vi "Measurement UI.vi"() -> ()   [LabVIEW 2021, in "Load Transient_Channel Ganging_UI.lvlib"]
uses:
  Load Transient_Channel Ganging_UI.lvlib
panel:
  in  "MeasGraphs":T1(tab)
  out "OutputCurrentV/STimeGraph":waveform(dbl)(graph) caption="Load Transient"
  in  "Load Current v/s Time":string="LOAD CURRENT vs TIME"
  in  "Output Voltage v/s Time":string="LOAD VOLTAGE vs TIME"
  out "OutputVoltageV/STimeGraph":waveform(dbl)(graph) caption="Load Transient"
  out "dt":dbl
  in  "Load current pole-zero ratio":dbl=0.3
  in  "Load current compensation frequency":dbl=180000.0
  in  "Load current gain bandwidth":dbl=14000.0
  in  "Source voltage pole-zero ratio":dbl=2.0
  in  "Source voltage compensation frequency":dbl=3530.0
  in  "Source voltage gain bandwidth":dbl=2000.0
  out "Ganged load voltages":dbl[](array[numeric])
  out "Ganged load current":dbl[](array[numeric])
  in  "Load slave resource names":string[](array[string])
  in  "Load master resource name":string
  in  "Source slave resource names":string[](array[string])
  in  "Source master resource name":string
  in  "MeasConfigurations":T2(tab)=enum."Source Config"
  in  "Nominal output voltage":dbl=1.0 caption="NOMINAL OUTPUT VOLTAGE" format="%.3pV"
  in  "DUT setup time":dbl=1.0 caption="DUT SETUP TIME" format="%.3ps"
  in  "Level dwell time":dbl=0.001 caption="DWELL TIME" format="%.3ps"
  in  "PPSSlaveResourceNames":refnum<k15>[](array[refnum]) caption="SLAVE RESOURCE NAMES"
  in  "PPSMasterResourceName":refnum<k15> caption="MASTER RESOURCE NAME"
  in  "Source transient response":i32(ring)=1038 caption="TRANSIENT RESPONSE" items=["Slow"=1041, "Normal"=1038, "Fast"=1039, "Custom"=1042]
  in  "Source sense":i32(ring)=1009 caption="SENSE" items=["Local"=1008, "Remote"=1009]
  in  "Source voltage level range":dbl=20.0 caption="VOLTAGE LEVEL RANGE" format="%#_6pV"
  in  "Source voltage level":dbl=12.0 caption="VOLTAGE LEVEL" format="%#_6pV"
  in  "Source current limit high":dbl=25.0 caption="CURRENT LIMIT/LIMIT HIGH" format="%#_6pA"
  in  "Source current limit range":dbl=25.0 caption="CURRENT LIMIT RANGE" format="%#_6pA"
  in  "Source limit symmetry":enum32{"Symmetric", "Asymmetric"}(ring)=enum."Asymmetric" caption="LIMIT SYMMETRY"
  in  "Source current limit low":dbl=-0.6 caption="CURRENT LIMIT LOW" format="%#_6pA"
  in  "Source system configuration":enum32{"Series", "Parallel"}(ring)=enum."Parallel" caption="SYSTEM CONFIG"
  in  "Source compliance":string="Compliance"
  in  "Source sourceadapt":string="SourceAdapt"
  in  "Source Custom Transient Response":bool
  in  "Load sample rate":dbl=1800000.0 caption="SAMPLE RATE" format="%#_6pS/s"
  in  "Load current set point 2":dbl=20.0 caption="CURRENT SET POINT 2" format="%#_6pA"
  in  "Load current set point 1":dbl=1.0 caption="CURRENT SET POINT 1" format="%#_6pA"
  in  "Load sourceadapt":string="SourceAdapt"
  in  "Load compliance":string="Compliance"
  in  "Load system configuration":enum32{"Series", "Parallel"}(ring)=enum."Parallel" caption="SYSTEM CONFIG"
  in  "Load voltage limit low":dbl caption="VOLTAGE  LIMIT LOW" format="%#_6pV"
  in  "Load limit symmetry":enum32{"Symmetric", "Asymmetric"}(ring) caption="LIMIT SYMMETRY"
  in  "Load voltage limit range":dbl=6.0 caption="VOLTAGE LIMIT RANGE" format="%#_6pV"
  in  "Load voltage limit high":dbl=inf caption="VOLTAGE LIMIT/LIMIT HIGH" format="%#_6p"
  in  "Load current level range":dbl=80.0 caption="CURRENT LEVEL RANGE" format="%#_6pA"
  in  "Load sense":i32(ring)=1009 caption="SENSE" items=["Local"=1008, "Remote"=1009]
  in  "Load transient response":i32(ring)=1038 caption="TRANSIENT RESPONSE" items=["Slow"=1041, "Normal"=1038, "Fast"=1039, "Custom"=1042]
  in  "LoadSlaveResourceNames":refnum<k15>[](array[refnum]) caption="SLAVE RESOURCE NAMES"
  in  "LoadMasterResourceName":refnum<k15> caption="MASTER RESOURCE NAME"
  in  "Load Custom Transient Response":bool
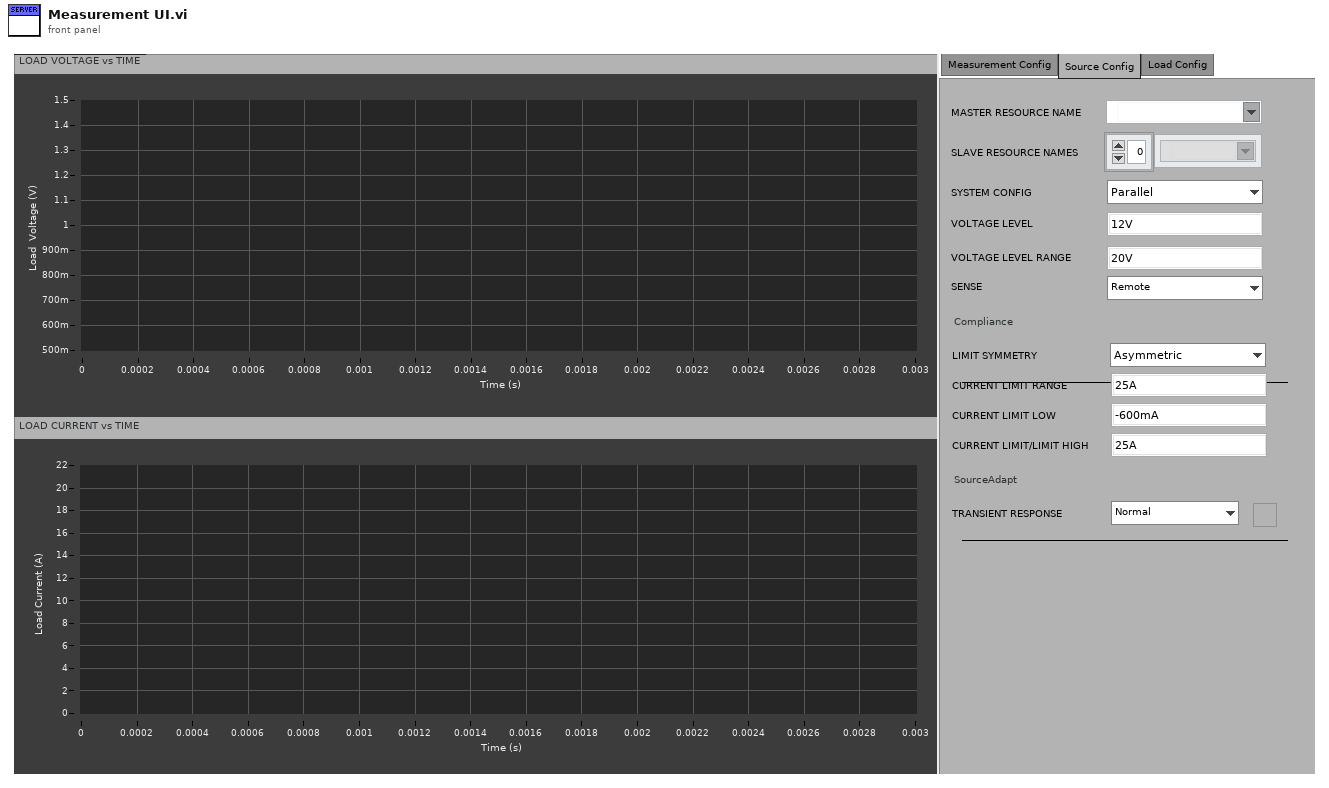
[diagram p1: front panel]
types:
  T1 = enum32{"Load transient response", "Hidden Controls"}
  T2 = enum32{"Measurement Config", "Source Config", "Load Config"}
  T3 = typedef "SourceAdapt Parameters.ctl" = cluster{"Voltage gain bandwidth":dbl, "Voltage compensation frequency":dbl, "Voltage pole-zero ratio":dbl, "Current gain bandwidth":dbl, "Current compensation frequency":dbl, "Current pole-zero ratio":dbl}
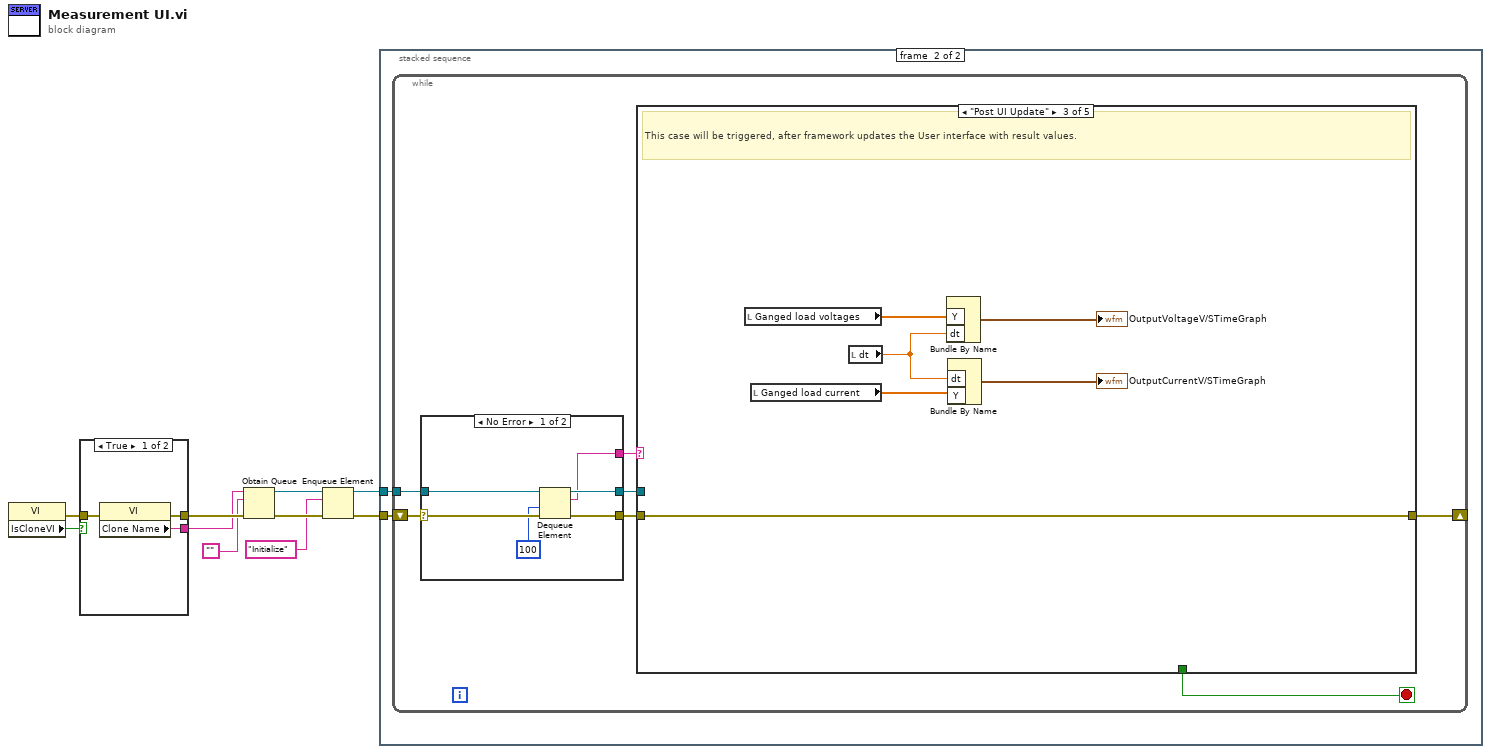
[diagram p0: block diagram]
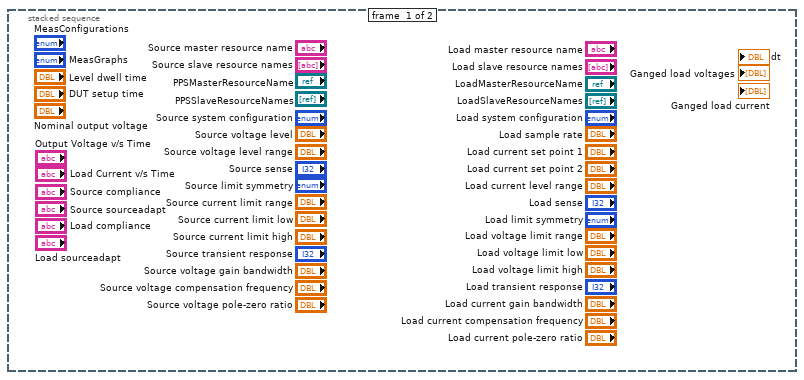
[diagram p2: hidden frame]
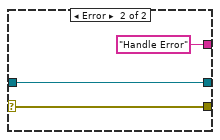
[diagram p3: hidden frame]
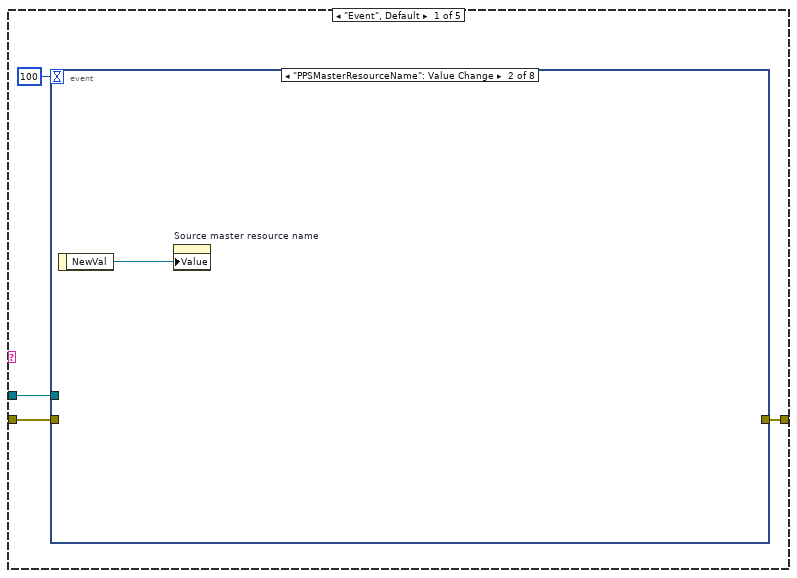
[diagram p4: hidden frame]
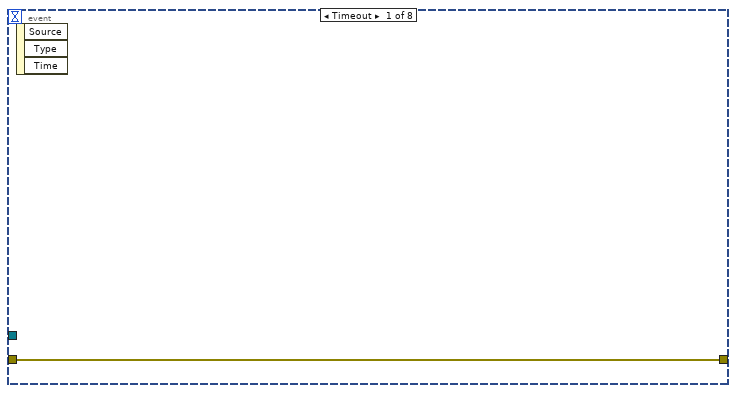
[diagram p5: hidden frame]
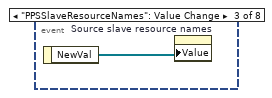
[diagram p6: hidden frame]
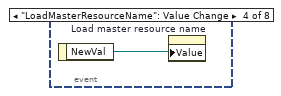
[diagram p7: hidden frame]
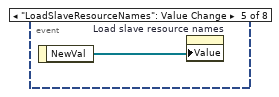
[diagram p8: hidden frame]
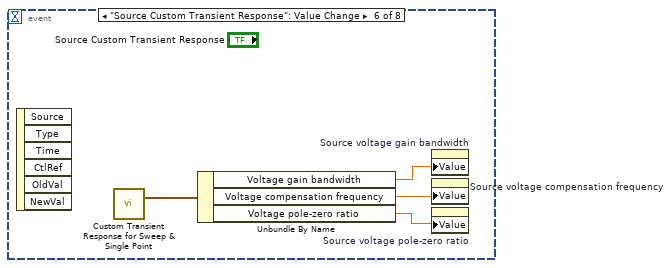
[diagram p9: hidden frame]
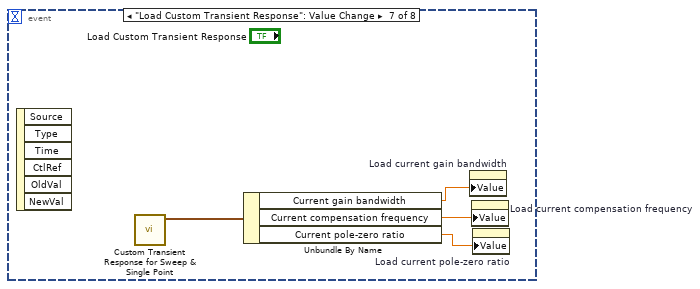
[diagram p10: hidden frame]
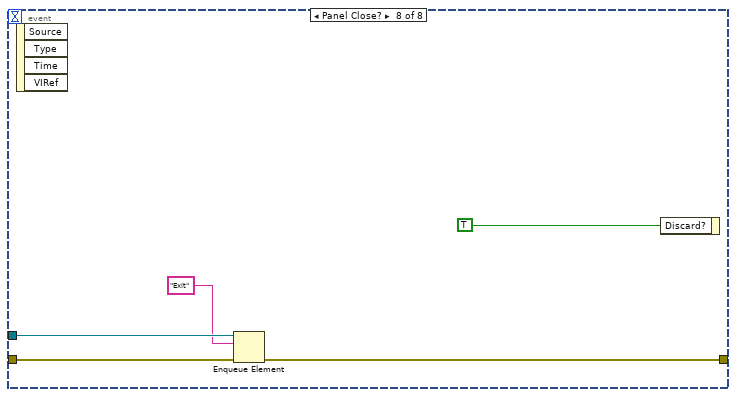
[diagram p11: hidden frame]
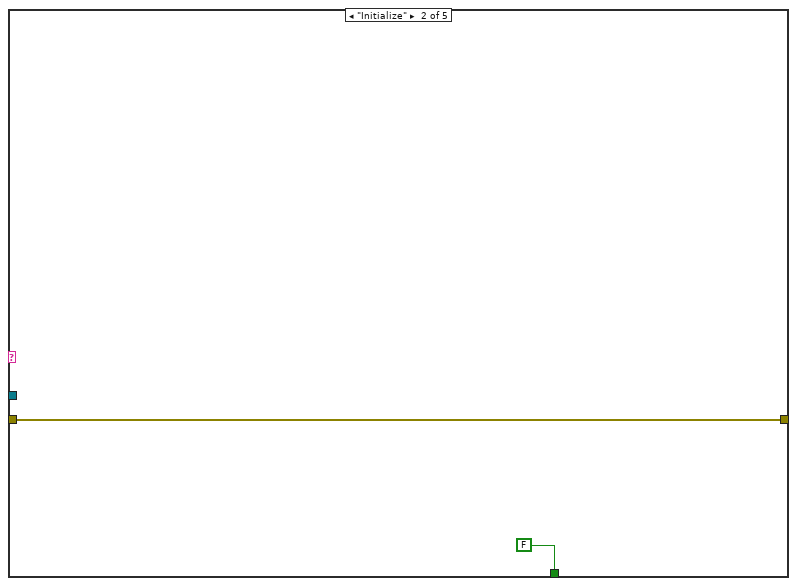
[diagram p12: hidden frame]
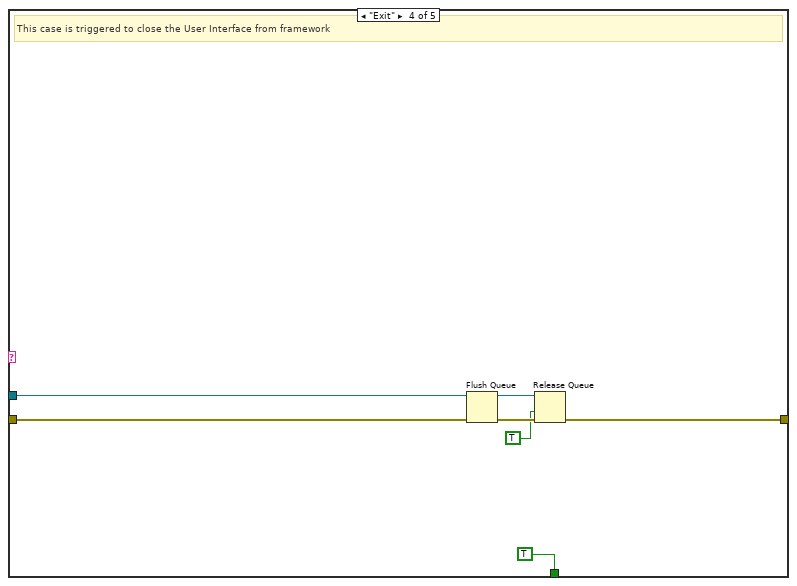
[diagram p13: hidden frame]
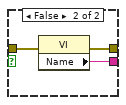
[diagram p15: hidden frame]
diagram:
  n1 = property class="VI"() -> (error out=w1:errorcluster, "IsCloneVI"=w2:bool)  [unwired: 2 in, 1 out]
  n2 = case shown="True" w2 {
    tunnel: [w13 w16] -> w10
    tunnel: [w12 w15] -> w9
    tunnel: w1 -> [w11 w14]
    frame True {
      n3 = property class="VI"(error in=w11) -> (error out=w13:errorcluster, "Clone Name"=w12:string)  [unwired: 1 in, 1 out]
    }
    frame False {
      n4 = property class="VI"(error in=w14) -> (error out=w16:errorcluster, "Name"=w15:string)  [unwired: 1 in, 1 out]
    }
  }
  n5 = Obtain Queue(name (unnamed)=w9, element data type="", error in (no error)=w10) -> (queue out=w6:refnum<queue>, error out=w8:errorcluster)  [unwired: 2 in, 1 out]
  n6 = Enqueue Element(queue=w6, element="Initialize", error in (no error)=w8) -> (queue out=w5:refnum<queue>, error out=w7:errorcluster)  [unwired: 1 in, 1 out]
  n7 = stacked-sequence {
    tunnel: w7 -> [_ w18]
    tunnel: w5 -> [_ w17]
    frame #0 {
    }
    frame #1 {
      n8 = while {
        shift-right: [w20] -> _
        shift-left: w18 -> [w25]
        tunnel: w17 -> [w23]
        stop <- w19 stop-if-true
        n9 = case shown="No Error" w25 {
          selector: w25 -> [w31 w34]
          tunnel: [w30 w34] -> w24
          tunnel: w23 -> [w29 w33]
          tunnel: [w28 w33] -> w22
          tunnel: [w27 "Handle Error"] -> w21
          frame No Error {
            n10 = Dequeue Element(queue=w29, timeout in ms (-1)=100, error in (no error)=w31) -> (queue out=w28:refnum<queue>, element=w27:string, error out=w30:errorcluster)  [unwired: 1 out]
          }
          frame Error {
          }
        }
        n11 = case shown="\"Post UI Update\"" w21 {
          tunnel: w24 -> [w37 w58 w64 w71 w72]
          tunnel: w22 -> [w35 _ _ w69 _]
          tunnel: [w38 w58 w64 w66 w72] -> w20
          tunnel: [_ FALSE _ TRUE _] -> w19
          frame "Event", Default {
            n12 = event shown="[1] \"PPSMasterResourceName\": Value Change" {
              selector: _ -> [_ _ _ _ _ _ _ _]
              dyn-events: _ -> [_ _ _ _ _ _ _ _]
              timeout: 100 -> [_ _ _ _ _ _ _ _]
              tunnel: [w39 _ _ _ _ _ _ w54] -> w38
              tunnel: w37 -> [w39 _ _ _ _ _ _ w55]
              tunnel: w35 -> [_ _ _ _ _ _ _ w53]
              event Timeout {
                n13 = event-data() -> ()  [unwired: 1 in, 3 out]
              }
              event "PPSMasterResourceName": Value Change {
                n14 = event-data() -> ("NewVal"=w40:refnum<k15>)  [unwired: 1 in]
                n15 = property on="Source master resource name" class="Str"("Value"=w40) -> ()  [unwired: 2 in, 2 out]
              }
              event "PPSSlaveResourceNames": Value Change {
                n16 = event-data() -> ("NewVal"=w41:refnum<k15>[])  [unwired: 1 in]
                n17 = property on="Source slave resource names" class="Arr (strict)"("Value"=w41) -> ()  [unwired: 2 in, 2 out]
              }
              event "LoadMasterResourceName": Value Change {
                n18 = event-data() -> ("NewVal"=w42:refnum<k15>)  [unwired: 1 in]
                n19 = property on="Load master resource name" class="Str"("Value"=w42) -> ()  [unwired: 2 in, 2 out]
              }
              event "LoadSlaveResourceNames": Value Change {
                n20 = event-data() -> ("NewVal"=w43:refnum<k15>[])  [unwired: 1 in]
                n21 = property on="Load slave resource names" class="Arr (strict)"("Value"=w43) -> ()  [unwired: 2 in, 2 out]
              }
              event "Source Custom Transient Response": Value Change {
                n22 = event-data() -> ()  [unwired: 1 in, 6 out]
                n23 = call "Custom Transient Response for Sweep & Single Point.vi"() -> ("SourceAdapt Parameters"=w47:T3)  [unwired: 11 in]
                n24 = Unbundle By Name(w47) -> ("Voltage gain bandwidth"=w46:dbl, "Voltage compensation frequency"=w45:dbl, "Voltage pole-zero ratio"=w44:dbl)
                n25 = property on="Source voltage gain bandwidth" class="DigNum (strict)"("Value"=w46) -> ()  [unwired: 2 in, 2 out]
                n26 = property on="Source voltage compensation frequency" class="DigNum (strict)"("Value"=w45) -> ()  [unwired: 2 in, 2 out]
                n27 = property on="Source voltage pole-zero ratio" class="DigNum (strict)"("Value"=w44) -> ()  [unwired: 2 in, 2 out]
              }
              event "Load Custom Transient Response": Value Change {
                n28 = event-data() -> ()  [unwired: 1 in, 6 out]
                n29 = call "Custom Transient Response for Sweep & Single Point.vi"() -> ("SourceAdapt Parameters"=w51:T3)  [unwired: 11 in]
                n30 = Unbundle By Name(w51) -> ("Current gain bandwidth"=w50:dbl, "Current compensation frequency"=w49:dbl, "Current pole-zero ratio"=w48:dbl)
                n31 = property on="Load current gain bandwidth" class="DigNum (strict)"("Value"=w50) -> ()  [unwired: 2 in, 2 out]
                n32 = property on="Load current compensation frequency" class="DigNum (strict)"("Value"=w49) -> ()  [unwired: 2 in, 2 out]
                n33 = property on="Load current pole-zero ratio" class="DigNum (strict)"("Value"=w48) -> ()  [unwired: 2 in, 2 out]
              }
              event Panel Close? {
                n34 = event-data() -> ()  [unwired: 1 in, 4 out]
                n35 = Enqueue Element(queue=w53, element="Exit", error in (no error)=w55) -> (error out=w54:errorcluster)  [unwired: 1 in, 2 out]
                n36 = event-data("Discard?"=TRUE) -> ()  [unwired: 1 in, 1 out]
              }
            }
          }
          frame "Initialize" {
          }
          frame "Post UI Update" {
            # "This case will be triggered, after framework updates the User interface with result values."
            n37 = local read "Ganged load voltages"() -> (w59:dbl[])
            n38 = local read "Ganged load current"() -> (w61:dbl[])
            n39 = local read "dt"() -> (w60:dbl)
            n40 = Bundle By Name("Y"=w59, "dt"=w60) -> (→"OutputVoltageV/STimeGraph":waveform(dbl))  [unwired: 1 in]
            n41 = Bundle By Name("dt"=w60, "Y"=w61) -> (→"OutputCurrentV/STimeGraph":waveform(dbl))  [unwired: 1 in]
          }
          frame "Exit" {
            # "This case is triggered to close the User Interface from framework"
            n42 = Flush Queue(queue=w69, error in (no error)=w71) -> (queue out=w68:refnum<queue>, error out=w67:errorcluster)  [unwired: 1 out]
            n43 = Release Queue(queue=w68, force destroy? (F)=TRUE, error in (no error)=w67) -> (error out=w66:errorcluster)  [unwired: 2 out]
          }
          frame "Handle Error" {
          }
        }
      }
    }
  }
